vi "Get Resource ID.vi"(4 "SPI CS in":refnum<class "SPI CS.lvclass">) -> (7 "Resource ID":string)   [LabVIEW 2024, in "CTI.lvlib" / "SPI CS.lvclass"]
uses:
  SPI CS.lvclass
  SPI CS.lvclass/SPI CS.ctl
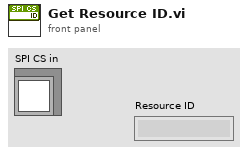
[diagram p1: front panel]
types:
  T1 = typedef "CTI.lvlib/GPIO Number.ctl" = i8
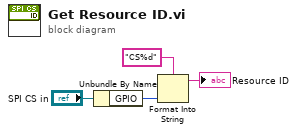
[diagram p0: block diagram]
diagram:
  n1 = Unbundle By Name("SPI CS in") -> ("GPIO"=w3:T1)
  n2 = Format Into String(format string="CS%d", w3) -> (resulting string=→"Resource ID":string)  [unwired: 2 in, 1 out]
